vi "LakeShore 336 curve.vi"(2 "error in (no error)":errorcluster, 3 "Curve Data Format 4: Log Ohms/K)":u16(ring)=4 items=["mV/K"=1, "V/K"=2, "Ohms/K"=3, "Log Ohms/K"=4], 4 "Curve":i32=21 min=21 max=59 step=1, 5 "VISA session":refnum<visa-resource-name>) -> (0 "error out":errorcluster, 1 "dup VISA session":refnum<visa-resource-name>)   [LabVIEW 2021]
doc: "This VI will upload a calibration curve to the LakeShore 336 Temperature Controller. It reads the data from a file and then formats it for uploading.\nJonathan Billings, <billings@magnet.fsu.edu> NHMFL-FSU, April 2010\n\nCode adapted from LakeShore 370 curve.vi\nScott Hannahs, <sth@magnet.fsu.edu> NHMFL-FSU, May 2003"
uses:
  Misc Extras/Manufacturer Drivers/LakeShore/Lake Shore Cryotronics 336/Lake Shore 336.lvlib
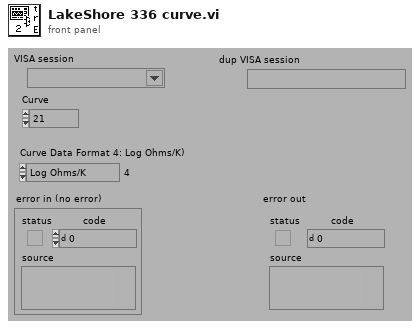
[diagram p1: front panel]
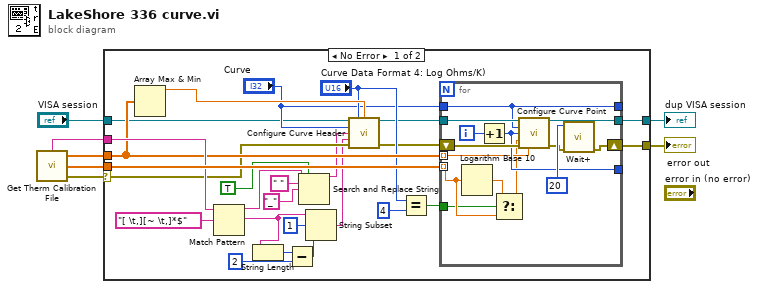
[diagram p0: block diagram]
diagram:
  n1 = call "Get Therm Calibration File.vi"() -> ("Calbration Name"=w6:string, "Temperature"=w5:dbl[], "Resistance"=w7:dbl[], "error out"=w1:errorcluster)  [unwired: 1 in]
  n2 = case shown="No Error" w1 {
    selector: w1 -> [w16 w48]
    tunnel: w7 -> [w33 _]
    tunnel: w6 -> [w30 _]
    tunnel: w5 -> [w25 _]
    tunnel: "VISA session" -> [w19 w49]
    tunnel: [w24 w48] -> w3
    tunnel: [w23 w49] -> w2
    frame No Error {
      n3 = Array Max & Min(array=w25) -> (max value=w22:dbl)  [unwired: 3 out]
      n4 = Match Pattern(string=w30, regular expression="[ \t,][~ \t,]*$") -> (before substring=w11:string, match substring=w8:string)  [unwired: 1 in, 2 out]
      n5 = String Length(string=w8) -> (length=w28:i32)
      n6 = Subtract(x=w28, y=2) -> (x-y=w26:i32)
      n7 = Search and Replace String(replace all?=TRUE ("replace all? (F)"), input string=w11, search string=" ", replace string="_" ("replace string (\"\")")) -> (result string=w10:string)  [unwired: 4 in, 3 out]
      n8 = String Subset(string=w8, offset (0)=1, length (rest)=w26) -> (substring=w14:string)
      n9 = call "Configure Curve Header.vi"("VISA resource name"=w19, "Curve Data Format (1:mV/K)"="Curve Data Format 4: Log Ohms/K)", "Limit Value (375.000)"=w22, "Curve (21)"="Curve", "Curve Name (\"\")"=w10, "Curve Serial Number (\"\")"=w14, "error in (no error)"=w16) -> ("VISA resource name out"=w18:refnum<visa-resource-name>, "error out"=w17:errorcluster)  [unwired: 7 in]
      n10 = Equal?(x="Curve Data Format 4: Log Ohms/K)", y=u16 4) -> (x = y?=w15:bool)
      n11 = for {
        tunnel: w25 -> [w35] mode=indexing
        tunnel: w33 -> [w45] mode=indexing
        tunnel: w18 -> [w41]
        tunnel: "Curve" -> [w37]
        tunnel: w15 -> [w44]
        tunnel: [w40] -> w23
        tunnel: [w36] -> _
        tunnel: [w37] -> _
        shift-right: [w43] -> w24
        shift-left: w17 -> [w39]
        i -> [w47]
        n12 = Logarithm Base 10(1:w45) -> (0:w46:dbl)
        n13 = Increment(x=w47) -> (x+1=w36:i32)
        n14 = Select(t=w46, s=w44, f=w45) -> (s? t:f=w34:dbl)
        n15 = call "Configure Curve Point.vi"("VISA resource name"=w41, "Curve (21)"=w37, "Index (1)"=w36, "Units Value (0.00000)"=w34, "error in (no error)"=w39, "Temperature Value (0.0000)"=w35) -> ("VISA resource name out"=w40:refnum<visa-resource-name>, "error out"=w38:errorcluster)  [unwired: 8 in]
        n16 = call "Wait+.vi"("Error In"=w38, "milliseconds to wait"=u32 20) -> ("Error Out"=w43:errorcluster)  [unwired: 4 in, 1 out]
      }
    }
    frame Error {
    }
  }
  "error out" <- w3
  "dup VISA session" <- w2
